vi "sv_Check for Weighting Conflict (N Ch).vi"(6 "weighting":T1 items=["Linear", "A-weighting", "B-weighting", "C-weighting", "ITU-R 468-4", "Dolby", "CCITT", "C-message", "Wb", "Wc", "Wd", "We", "Wf", "Wh", "Wj", "Wk", "Wm", "AES17 20 kHz lowpass", "AES17 40 kHz lowpass", "AES17 20 kHz highpass", "AES17 40 kHz highpass"], 8 "error in (no error)":errorcluster, 11 "scaled signals":waveform(dbl)[](array[waveform])) -> (0 "error out":errorcluster, 3 "dup scaled signals":waveform(dbl)[](array[waveform]), 4 "weighting":T1 items=["Linear", "A-weighting", "B-weighting", "C-weighting", "ITU-R 468-4", "Dolby", "CCITT", "C-message", "Wb", "Wc", "Wd", "We", "Wf", "Wh", "Wj", "Wk", "Wm", "AES17 20 kHz lowpass", "AES17 40 kHz lowpass", "AES17 20 kHz highpass", "AES17 40 kHz highpass"])   [LabVIEW 2017]
doc: "Make sure we will not be applying weighting twice if an external weighting filter has been used"
uses:
  <vilib>/addons/_NISVFA/_Shared subVIs/Controls/svc_Weighting Filter Text Ring.ctl
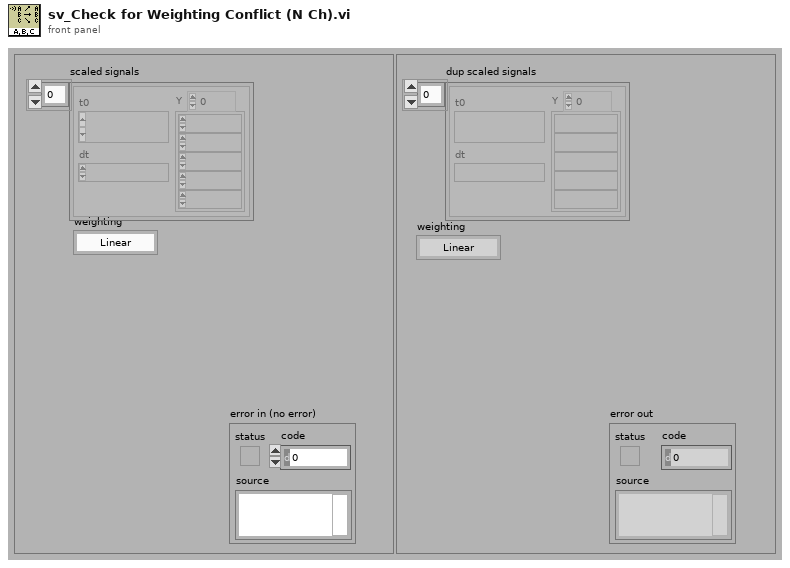
[diagram p1: front panel]
types:
  T1 = typedef "svc_Weighting Filter Text Ring.ctl" = u16
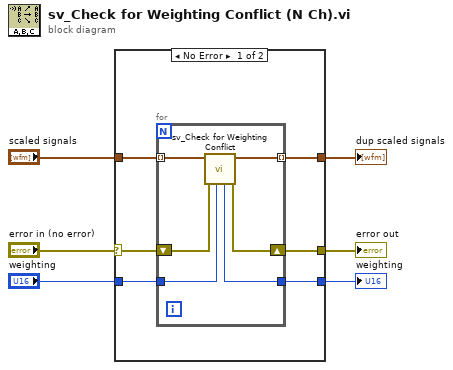
[diagram p0: block diagram]
diagram:
  n1 = case shown="No Error" "error in (no error)" {
    selector: "error in (no error)" -> [w11 w19]
    tunnel: "scaled signals" -> [w12 w21]
    tunnel: [w10 w21] -> w4
    tunnel: "weighting" -> [w9 w20]
    tunnel: [w8 w20] -> w2
    tunnel: [w7 w19] -> w1
    frame No Error {
      n2 = for {
        shift-right: [w16] -> w7
        shift-left: w11 -> [w15]
        tunnel: w12 -> [w18] mode=indexing
        tunnel: [w17] -> w10 mode=indexing
        tunnel: w9 -> [w14]
        tunnel: [w13] -> w8
        n3 = call <vilib>:"sv_Check for Weighting Conflict.vi"("weighting"=w14, "error in (no error)"=w15, "scaled signal [EU]"=w18) -> ("error out"=w16:errorcluster, "scaled signal [EU]"=w17:waveform(dbl), "dup weighting"=w13:T1)  [unwired: 6 in]
      }
    }
    frame Error {
    }
  }
  "error out" <- w1
  "weighting" <- w2
  "dup scaled signals" <- w4
